vi "assertTrigger.vi"(7 "address":string, 8 "error in (no error)":errorcluster, 11 "Trigger":bool=TRUE) -> (0 "error out":errorcluster)   [LabVIEW 2016]
doc: "API to assert the trigger.\n\nIf address=\"\", this API reads from localhost\nIf address is remote lockin, you need to add this computer to allowed whitelist on the lockin computer you are trying to access."
uses:
  SMOs/RemoteControl/Typedefs/Remote-SMO-Commands-Enum.ctl
  <vilib>/addons/_JKI.lib/Serialization/JSON/JKI JSON Serialization.lvlib
  SMOs/RemoteControl/RemoteControl.lvclass
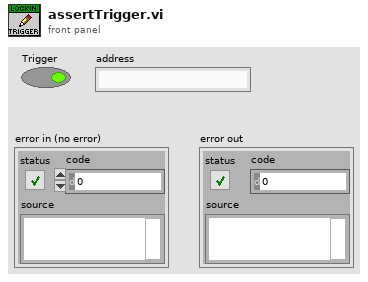
[diagram p1: front panel]
types:
  T1 = typedef "RemoteControl.lvclass/Remote-SMO-Commands-Enum.ctl" = enum16{"configAO", "configREF", "configIVmode", "configRemote", "configReset", "assertTrigger", "getAO", "getAI", "getResults", "getTrigger", "getIVmode", "getAOconfig", "getREFconfig", "ACK", "UNK", "CLOSE"}
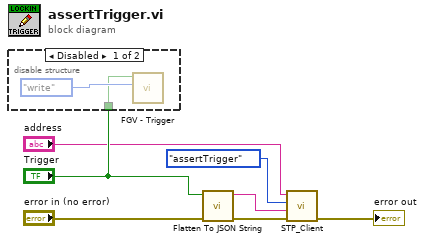
[diagram p0: block diagram]
diagram:
  n1 = disable-structure shown="Disabled" {
    disable-tunnel: "Trigger" -> [w8 _]
    frame Disabled {
      n2 = call "FGV - Trigger.vi"("Function"=enum16{"write", "read"}."write", "Trigger"=w8) -> ()  [unwired: 4 in, 2 out]
    }
    frame Enabled {
    }
  }
  n3 = call <vilib>:"Flatten To JSON String.vi"("error in (no error)"="error in (no error)", "Variant"="Trigger") -> ("error out"=w6:errorcluster, "JSON String"=w5:string)  [unwired: 8 in]
  n4 = call "STP_Client.vi"("error in (no error)"=w6, "data to send"=w5, "Command"=Remote-SMO-Commands-Enum."assertTrigger", "address"="address") -> ("error out"=→"error out":errorcluster)  [unwired: 6 in, 1 out]
